vi "FTW-SQLite-Core-LibraryReturnValue.vi"(0 "error in":errorcluster, 7 "Return Value":i32) -> (4 "error out":errorcluster)   [LabVIEW 2015]
uses:
  error/FTW-ERR-CallChain.vi
  error/FTW-ERR-NoErrorConstant.vi
  string/FTW-STR-ReplaceWhitespace.vi
  string/FTW-STR-Array-Delimit.vi
  error/FTW-ERR-Clear.vi
  regex/FTW-Regex-ReplaceAll.vi
panel:
  # "Inputs"
  # "Outputs"
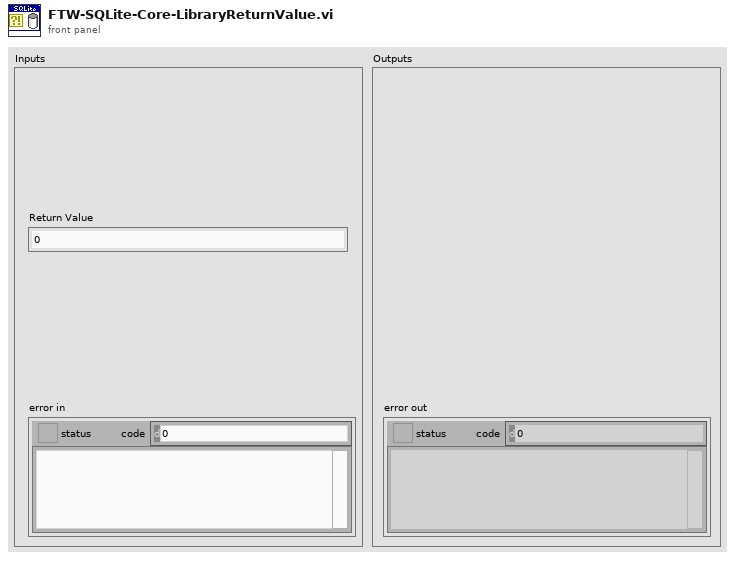
[diagram p1: front panel]
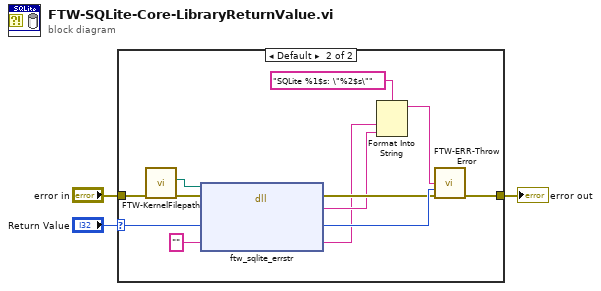
[diagram p0: block diagram]
diagram:
  n1 = case shown="Default" "Return Value" {
    selector: "Return Value" -> [_ w10]
    tunnel: "error in" -> [w4 w6]
    tunnel: [w4 w16] -> w2
    frame 0 {
    }
    frame Default {
      n2 = call "FTW-KernelFilepath.vi"("error in"=w6) -> ("error out"=w5:errorcluster, "Library Filepath"=w7:path)  [unwired: 8 in, 1 out]
      n3 = dll-call lib="?" fn="ftw_sqlite_errstr"(path in=w7, error in=w5, "Error Code"=w10, "Library Version"="") -> (error out=w12:errorcluster, "Error Message"=w11:string, "Error Code"=w13:i32, "Library Version"=w8:string)  [unwired: 1 in, 1 out]
      n4 = Format Into String(format string="SQLite %1$s: \"%2$s\"" ("Error Message"), w8, w11) -> (resulting string=w14:string)  [unwired: 2 in, 1 out]
      n5 = call "FTW-ERR-ThrowError.vi"("Error Message"=w14, "Error Code"=w13, "error in"=w12) -> ("error out"=w16:errorcluster)  [unwired: 12 in]
    }
  }
  "error out" <- w2
